vi "Adjust cosmetics for co-ordinate system.vi"(5 "Ring Refnum In":refnum<vi>, 7 "TabCtl Refnum In":refnum<vi>, 8 "Error In (no Error) In":errorcluster, 9 "Coordinate System In":bool, 11 "Display State In":T1 caption="State") -> (0 "Error In (no Error) Out":errorcluster, 3 "Display State Out":T1 caption="State")   [LabVIEW 2018, in "Vector Function Generator.xctl"]
doc: "Update the labels on controls to match the switch between polar and cartesian modes"
uses:
  Vector Function Generator.xctl
  Vector State.ctl
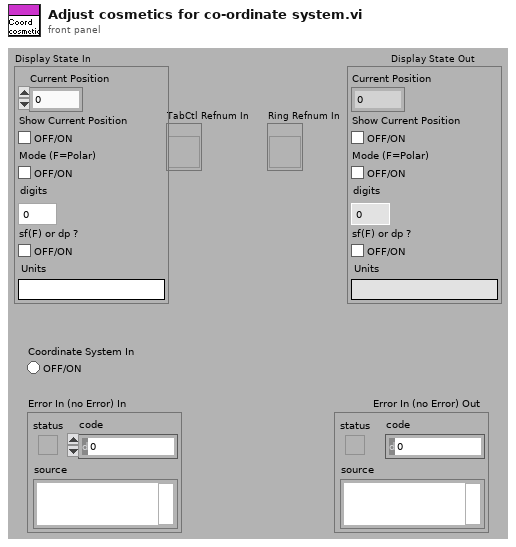
[diagram p1: front panel]
types:
  T1 = typedef "Vector Function Generator.xctl/Vector State.ctl" = cluster{"Current Position":i32, "Show Current Position":bool, "Mode (F=Polar)":bool, "digits":i32, "sf(F) or dp ?":bool, "Units":string}
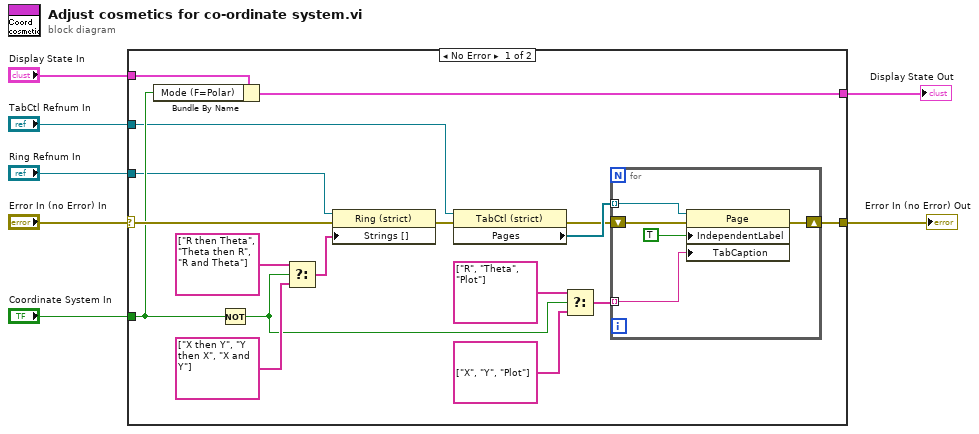
[diagram p0: block diagram]
diagram:
  n1 = case shown="No Error" "Error In (no Error) In" {
    selector: "Error In (no Error) In" -> [w23 w31]
    tunnel: [w24 w31] -> w7
    tunnel: "Coordinate System In" -> [w22 _]
    tunnel: [w21 w30] -> w4
    tunnel: "Display State In" -> [w20 w30]
    tunnel: "TabCtl Refnum In" -> [w19 _]
    tunnel: "Ring Refnum In" -> [w18 _]
    frame No Error {
      n2 = Bundle By Name(cluster=w20, "Mode (F=Polar)"=w22) -> (w21:T1)
      n3 = Not(x=w22) -> (.not. x?=w11:bool)
      n4 = Select(t=string[] ["R then Theta", "Theta then R", "R and Theta"] ("item names"), s=w11, f=string[] ["X then Y", "Y then X", "X and Y"] ("item names")) -> (s? t:f=w12:string[])
      n5 = property on="Property Node" class="Ring (strict)"(reference=w18, error in=w23, "Strings []"=w12) -> (error out=w8:errorcluster)  [unwired: 1 out]
      n6 = property on="Property Node" class="TabCtl (strict)"(reference=w19, error in=w8) -> (error out=w9:errorcluster, "Pages"=w10:refnum<vi>[])  [unwired: 1 out]
      n7 = Select(t=string[] ["R", "Theta", "Plot"] ("item names"), s=w11, f=string[] ["X", "Y", "Plot"] ("item names")) -> (s? t:f=w15:string[])
      n8 = for {
        tunnel: w10 -> [w29] mode=indexing
        tunnel: w15 -> [w28] mode=indexing
        shift-right: [w25] -> w24
        shift-left: w9 -> [w26]
        n9 = property class="Page"(reference=w29, error in=w26, "IndependentLabel"=TRUE ("Independent Label"), "TabCaption"=w28) -> (error out=w25:errorcluster)  [unwired: 1 out]
      }
    }
    frame Error {
    }
  }
  "Error In (no Error) Out" <- w7
  "Display State Out" <- w4
